vi "create navigational matrix.vi"(1 "parameters":T2(array[cluster]) {"angle" scale=0.0..6.283184}) -> (0 "Array":T1(array[cluster]))   [LabVIEW 2009]
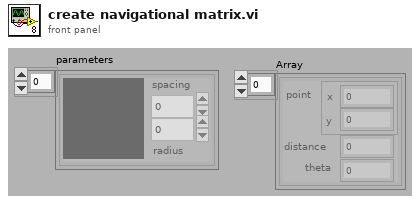
[diagram p1: front panel]
types:
  T1 = cluster{"point":cluster{"x":i16, "y":i16}, "distance":u16, "theta":dbl}[]
  T2 = cluster{"spacing":i16, "radius":u16, "angle":dbl}[]
  T3 = cluster{"point":cluster{"x":i16, "y":i16}, "radius":u16, dbl}[]
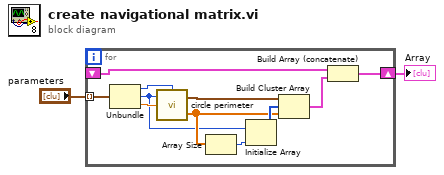
[diagram p0: block diagram]
diagram:
  n1 = for {
    tunnel: "parameters" -> [w13] mode=indexing
    shift-right: [w11] -> w1
    shift-left: _ -> [w12]
    n2 = Unbundle(w13) -> ("spacing"=w4:i16, "radius"=w3:u16, "angle"=w10:dbl)
    n3 = call "circle perimeter.vi"("spacing between points (1)"=w4, "arc start (radians)"=w10, "radius"=w3) -> ("theta"=w7:dbl[], "points along perimeter"=w9:cluster{"x":i16, "y":i16}[])  [unwired: 1 in]
    n4 = Array Size(array=w7) -> (size(s)=w6:i32)
    n5 = Initialize Array(w3, w6) -> (w8:u16[])
    n6 = Build Cluster Array(w9, w8, w7) -> (w5:T3)
    n7 = Build Array (concatenate)(w12, w5) -> (w11:T3)
  }
  "Array" <- w1
